vi "MoveSlide.vi"(1 "Target":path=path "/Kim/Users/crogers/Dropbox/LVPresent/Talk/Slides/test3.vi", 2 "Source":path=path "/Kim/Users/crogers/Dropbox/LVPresent/Templates/MovieTemplate.vi") -> (0 "Success?":bool=TRUE)   [LabVIEW 2014]
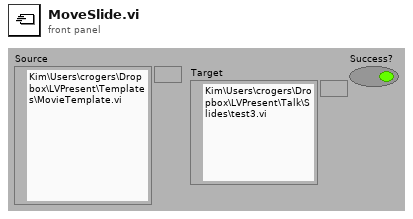
[diagram p1: front panel]
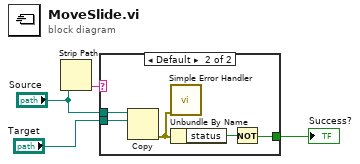
[diagram p0: block diagram]
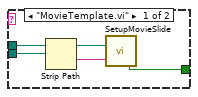
[diagram p2: hidden frame]
diagram:
  n1 = Strip Path(path="Source") -> (name=w1:string)  [unwired: 1 out]
  n2 = case shown="Default" w1 {
    tunnel: [w5 w12] -> w4
    tunnel: "Source" -> [w6 w10]
    tunnel: "Target" -> [w7 w9]
    frame "MovieTemplate.vi" {
      n3 = Strip Path(path=w7) -> (name=w8:string)  [unwired: 1 out]
      n4 = call "SetupMovieSlide.vi"("Name"=w8, "Template"=w6) -> ("success?"=w5:bool)
    }
    frame Default {
      n5 = Copy(10:w9, 11:w10) -> (0:w13:errorcluster)  [unwired: 3 in, 2 out]
      n6 = call <vilib>:"Simple Error Handler.vi"("error in (no error)"=w13) -> ()  [unwired: 4 in, 5 out]
      n7 = Unbundle By Name(w13) -> ("status"=w11:bool)
      n8 = Not(x=w11) -> (.not. x?=w12:bool)
    }
  }
  "Success?" <- w4
